vi "Send Switch Schedule Update.vi"(8 "error in (no error)":errorcluster, 11 "Switch Schedule":T1) -> (0 "error out":errorcluster)   [LabVIEW 2014]
doc: "Sends Switch Schedule updates to myRIO."
uses:
  myRIO/Controls/Switch Schedule.ctl
  myRIO/Controls/Switch Program.ctl
  myRIO/Controls/Action Enum.ctl
  myRIO/Controls/Switch Day.ctl
  Controls/UDP Reference Action Enum.ctl
panel:
  out "concatenated string":string
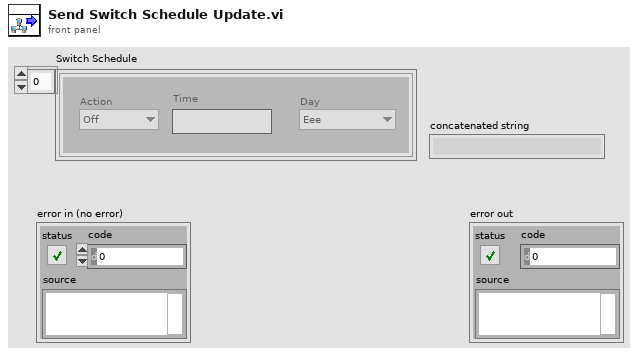
[diagram p1: front panel]
types:
  T1 = typedef "Switch Schedule.ctl" = T2[]
  T2 = typedef "Switch Program.ctl" = cluster{"Action":T3, "Time":string, "Day":T4}
  T3 = typedef "Action Enum.ctl" = enum16{"Off", "On"}
  T4 = typedef "Switch Day.ctl" = enum16{"Eee", "Sun", "Mon", "Tue", "Wed", "Thu", "Fri", "Sat"}
  T5 = typedef "UDP Reference Action Enum.ctl" = enum16{"Set", "Get"}
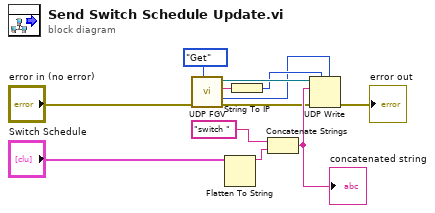
[diagram p0: block diagram]
diagram:
  n1 = call "UDP FGV.vi"("Action"=UDP_Reference_Action_Enum."Get", "error in (no error)"="error in (no error)") -> ("error out"=w8:errorcluster, "Port Out"=w3:u16, "IP Address out"=w5:string, "connection ID out"=w9:refnum<k16>)  [unwired: 6 in]
  n2 = Flatten To String(anything="Switch Schedule") -> (data string=w2:string)  [unwired: 3 in, 2 out]
  n3 = String To IP(1:w5) -> (0:w4:u32)
  n4 = Concatenate Strings("switch ", w2) -> (w12:string)
  "concatenated string" <- w12
  n5 = UDP Write(address=w4, port or service name=w3, connection ID=w9, data in=w12, 8:w8) -> (error out=→"error out":errorcluster)  [unwired: 1 in, 1 out]
